vi "Set Shutter.vi"(8 "error in":errorcluster, 10 "Shutter":bool, 11 "LTB-1 in":refnum<class "LTB-1.lvclass">) -> (0 "error out":errorcluster, 3 "LTB-1 out":refnum<class "LTB-1.lvclass">)   [LabVIEW 2018, in "LTB-1.lvlib" / "LTB-1.lvclass"]
doc: "This is a dynamically dispatched VI, the child method will build the appropriate message to send to the exfo to appropriately open or close the shutter for the optical load.\n\nAuthor: Ron Dexter\nCompany: Luminar\nModified: 5/20/2018"
uses:
  LTB-1.lvclass
  C:/AME Test Engineering/LabVIEW/PPLs/EXFO/Parent/EXFO.lvlibp/EXFO.lvclass
  LTB-1.lvclass/LTB-1.ctl
  PPLs/EXFO/Parent/EXFO.lvlibp/Methods/Read Resource.vi
  3150 Driver/3150.lvlib
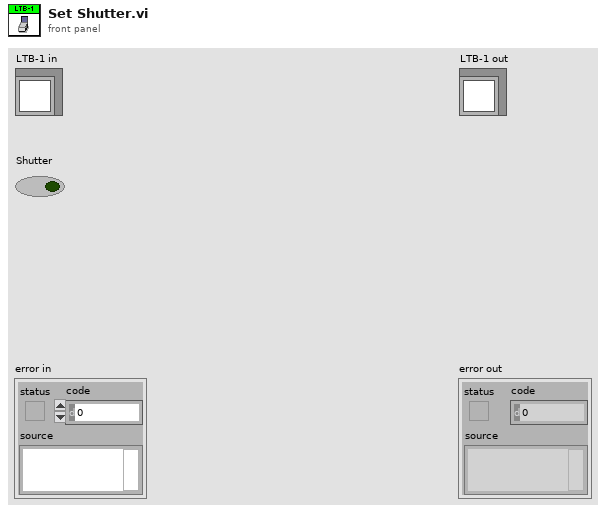
[diagram p1: front panel]
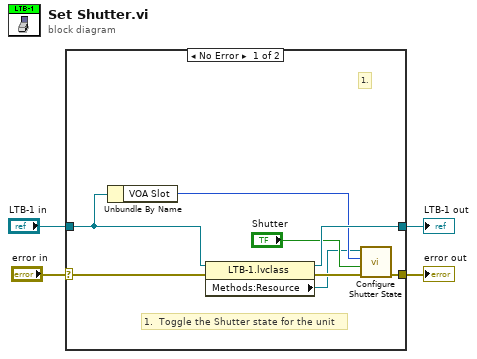
[diagram p0: block diagram]
diagram:
  n1 = case shown="No Error" "error in" {
    selector: "error in" -> [w11 w14]
    tunnel: "LTB-1 in" -> [w10 w13]
    tunnel: [w12 w13] -> w3
    tunnel: [w9 w14] -> w2
    frame No Error {
      # "1.  Toggle the Shutter state for the unit"
      # "1."
      n2 = Unbundle By Name(w10) -> ("VOA Slot"=w6:i16)
      n3 = property class="LTB-1.lvclass"(reference=w10, error in=w11) -> (reference out=w12:refnum<class "LTB-1.lvclass">, error out=w8:errorcluster, "Methods:Resource"=w5:refnum<visa-resource-name>)
      n4 = call "Configure Shutter State.vi"("error in (no error)"=w8, "Enable Shutter State (F:OFF)"="Shutter", "Platform Slot Number (10)"=w6, "VISA resource name"=w5) -> ("error out"=w9:errorcluster)  [unwired: 6 in, 1 out]
    }
    frame Error {
    }
  }
  "error out" <- w2
  "LTB-1 out" <- w3
